vi "DriveGetGyroIntDirection.vi"() -> (3 "GyroIntDirection":dbl)   [LabVIEW 2023]
doc: "Get GyroZero from drive for use elsewhere\n\nOutputs:\n-- GyroZero -- Double -- gets gyro zero from drive global"
uses:
  DriveGlobal.vi
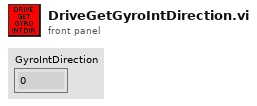
[diagram p1: front panel]
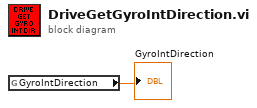
[diagram p0: block diagram]
diagram:
  n1 = global read "DriveGlobal.vi" "GyroIntDirection"() -> (→"GyroIntDirection":dbl)
